vi "CheesyVision.vi"(10 "No Hand Time":u32, 11 "Timeout":u32) -> (1 "No Connection":bool, 2 "No Hand":bool, 3 "Timeout":bool)   [LabVIEW 2013]
uses:
  Robot Global Data.vi
panel:
  out "Connected":bool
  out "Left":bool
  out "Right":bool
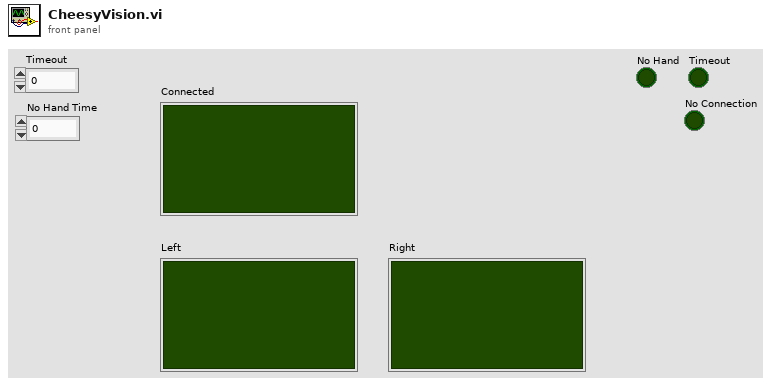
[diagram p1: front panel]
types:
  T1 = cluster{"Connected":bool, "Right":bool, "Left":bool}
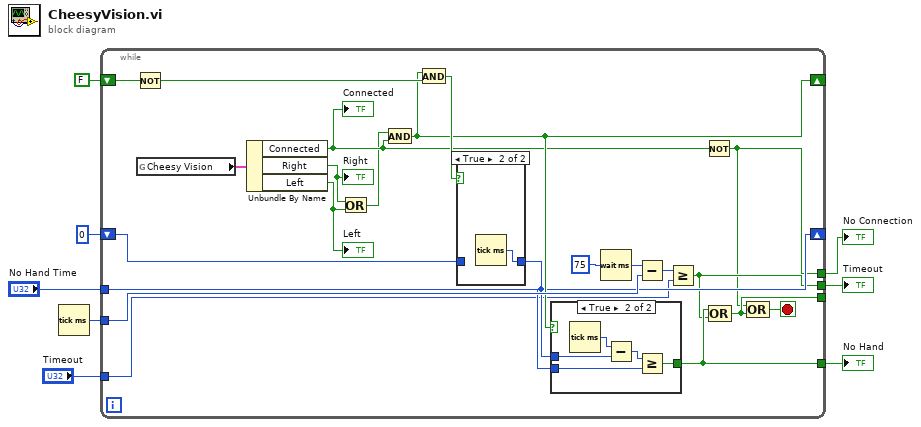
[diagram p0: block diagram]
diagram:
  n1 = Tick Count (ms)() -> (millisecond timer value=w2:u32)
  n2 = while {
    tunnel: [w19] -> _
    tunnel: w2 -> [w29]
    tunnel: "Timeout" -> [w20]
    shift-right: [w23] -> _
    shift-left: FALSE -> [w26]
    shift-right: [w22] -> _
    shift-left: u32 0 ("millisecond timer value") -> [w24]
    tunnel: "No Hand Time" -> [w21]
    tunnel: [w18] -> w6
    tunnel: [w17] -> w5
    tunnel: [w9] -> w4
    stop <- w16 stop-if-true
    n3 = Not(x=w26) -> (.not. x?=w27:bool)
    n4 = global read "Robot Global Data.vi" "Cheesy Vision"() -> (w15:T1)
    n5 = Unbundle By Name(w15) -> ("Connected"=w14:bool, "Right"=w12:bool, "Left"=w11:bool)
    "Right" <- w12
    "Left" <- w11
    "Connected" <- w14
    n6 = Or(x=w12, y=w11) -> (x .or. y?=w13:bool)
    n7 = And(x=w13, y=w14) -> (x .and. y?=w23:bool)
    n8 = And(x=w23, y=w27) -> (x .and. y?=w25:bool)
    n9 = case shown="True" w25 {
      tunnel: [w36 w37] -> w22
      tunnel: w24 -> [w36 _]
      frame False {
      }
      frame True {
        n10 = Tick Count (ms)() -> (millisecond timer value=w37:u32)
      }
    }
    n11 = case shown="True" w23 {
      tunnel: w22 -> [_ w33]
      tunnel: w21 -> [_ w32]
      tunnel: [_ w31] -> w18
      frame False {
      }
      frame True {
        n12 = Tick Count (ms)() -> (millisecond timer value=w34:u32)
        n13 = Subtract(x=w34, y=w33) -> (x-y=w35:u32)
        n14 = Greater Or Equal?(x=w35, y=w32) -> (x >= y?=w31:bool)
      }
    }
    n15 = Wait (ms)(milliseconds to wait=u32 75) -> (millisecond timer value=w30:u32)
    n16 = Subtract(x=w30, y=w29) -> (x-y=w28:u32)
    n17 = Greater Or Equal?(x=w28, y=w20) -> (x >= y?=w17:bool)
    n18 = Not(x=w14) -> (.not. x?=w9:bool)
    n19 = Compound Arithmetic op=OR(w18, w17) -> (w19:bool)
    n20 = Compound Arithmetic op=OR(w9, w19) -> (w16:bool)
  }
  "No Hand" <- w6
  "Timeout" <- w5
  "No Connection" <- w4
